vi "Dot_to_Comma.vi"(1 "String in":string) -> (0 "String out":string)   [LabVIEW 2018]
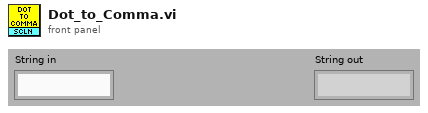
[diagram p1: front panel]
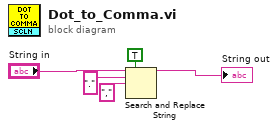
[diagram p0: block diagram]
diagram:
  n1 = Search and Replace String(replace all?=TRUE ("replace all? (F)"), input string="String in", search string=".", replace string="," ("replace string (\"\")")) -> (result string=→"String out":string)  [unwired: 1 in, 6 out]
